vi "UART_U8Read_Timeout.vi"(8 "error in (no error)":errorcluster caption="错误输入（无错误）", 9 "断帧时间ms":u32=10, 10 "超时s":dbl=0.1, 11 "BASE_COM":refnum<visa-resource-name>="COM1") -> (0 "error out":errorcluster caption="错误输出", 1 "HasDat":bool, 2 "Strout":string, 3 "BASE_COM_OUT":refnum<visa-resource-name>)   [LabVIEW 2015, in "UARTCOM.lvlib"]
uses:
  UARTCOM.lvlib
panel:
  # ">=10ms"
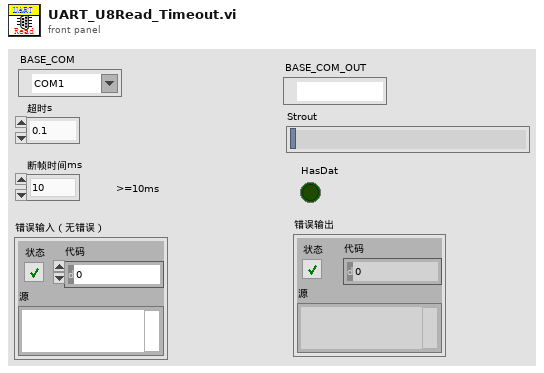
[diagram p1: front panel]
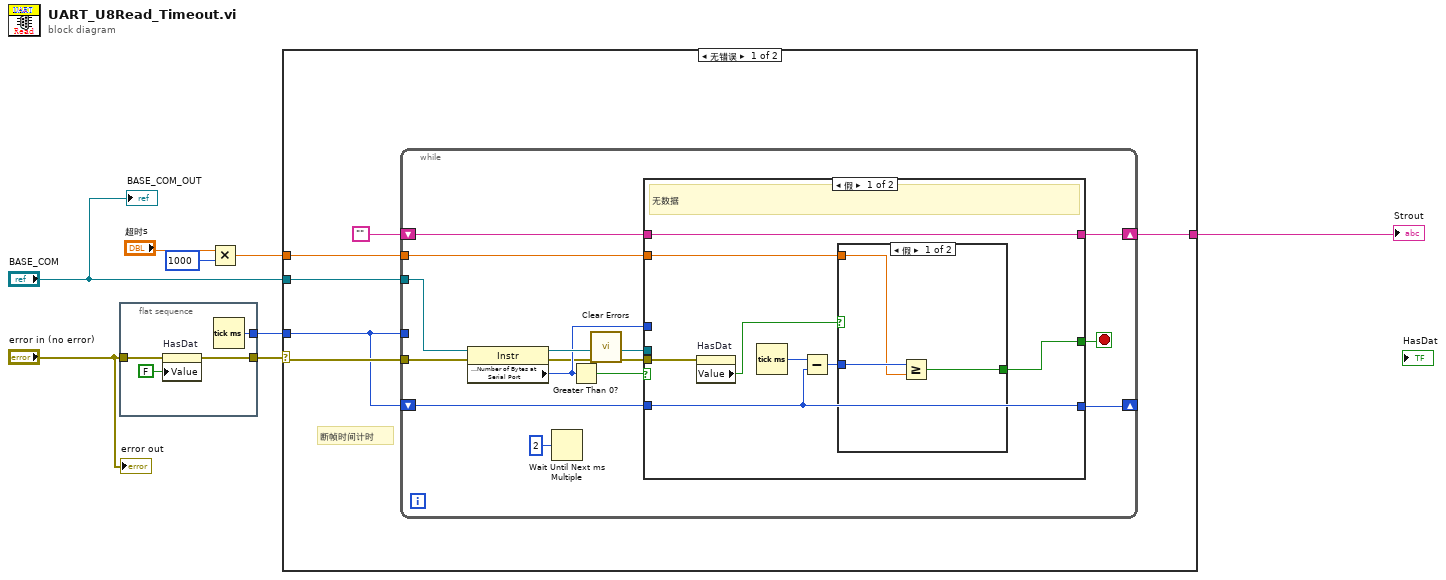
[diagram p0: block diagram]
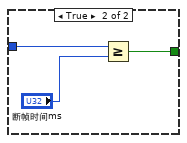
[diagram p2: hidden frame]
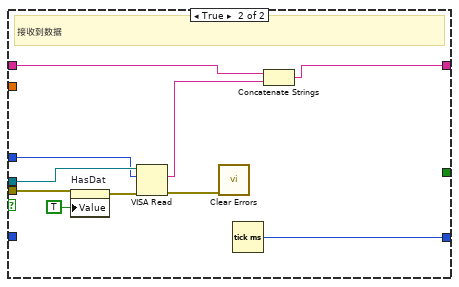
[diagram p3: hidden frame]
diagram:
  n1 = flat-sequence {
    tunnel: "error in (no error)" -> [w11]
    tunnel: [w10] -> w8
    tunnel: [w12] -> w7
    frame #0 {
      n2 = property on="HasDat" class="Bool (严格)"(error in=w11, "Value"=FALSE ("FirstIn")) -> (error out=w10:errorcluster)  [unwired: 1 in, 1 out]
      n3 = Tick Count (ms)() -> (millisecond timer value=w12:u32)
    }
  }
  n4 = Multiply(x="超时s", y=1000) -> (x*y=w4:dbl)
  n5 = case shown="无错误" w8 {
    selector: w8 -> [w17 _]
    tunnel: "BASE_COM" -> [w18 _]
    tunnel: w7 -> [w13 _]
    tunnel: w4 -> [w15 _]
    tunnel: [w14 _] -> w1
    frame No Error {
      # "断帧时间计时"
      n6 = while {
        tunnel: w18 -> [w32]
        tunnel: w17 -> [w31]
        tunnel: w13 -> [_]
        shift-right: [w24] -> w14
        shift-left: "" -> [w27]
        shift-right: [w28] -> _
        shift-left: w13 -> [w29]
        tunnel: w15 -> [w23]
        stop <- w22 stop-if-true
        n7 = property class="Instr"(reference=w32, error in=w31) -> (reference out=w26:refnum<visa-resource-name>, error out=w21:errorcluster, "Serial Settings:Number of Bytes at Serial Port"=w25:u32)
        n8 = Wait Until Next ms Multiple(millisecond multiple=u32 2 ("毫秒倍数")) -> ()  [unwired: 1 out]
        n9 = Greater Than 0?(x=w25) -> (x > 0?=w30:bool)
        n10 = call <vilib>:"Clear Errors.vi"("error in (no error)"=w21) -> ("error out"=w20:errorcluster)  [unwired: 5 in, 1 out]
        n11 = case shown="假" w30 {
          tunnel: w20 -> [w37 w56]
          tunnel: w29 -> [w39 _]
          tunnel: [w39 w54] -> w28
          tunnel: w27 -> [w38 w49]
          tunnel: w26 -> [_ w52]
          tunnel: w25 -> [_ w51]
          tunnel: [w38 w47] -> w24
          tunnel: w23 -> [w34 _]
          tunnel: [w33 _] -> w22
          frame False {
            # "无数据"
            n12 = property on="HasDat" class="Bool (严格)"(error in=w37) -> ("Value"=w36:bool)  [unwired: 1 in, 2 out]
            n13 = Tick Count (ms)() -> (millisecond timer value=w40:u32)
            n14 = Subtract(x=w40, y=w39) -> (x-y=w35:u32)
            n15 = case shown="假" w36 {
              tunnel: w35 -> [w43 w46]
              tunnel: w34 -> [w42 _]
              tunnel: [w41 w44] -> w33
              frame False {
                n16 = Greater Or Equal?(x=w43, y=w42) -> (x >= y?=w41:bool)
              }
              frame True {
                n17 = Greater Or Equal?(x=w46, y="断帧时间ms") -> (x >= y?=w44:bool)
              }
            }
          }
          frame True {
            # "接收到数据"
            n18 = property on="HasDat" class="Bool (严格)"(error in=w56, "Value"=TRUE ("FirstIn")) -> (error out=w53:errorcluster)  [unwired: 1 in, 1 out]
            n19 = VISA Read(VISA resource name=w52, byte count=w51, error in (no error)=w53) -> (read buffer=w48:string, error out=w50:errorcluster)  [unwired: 2 out]
            n20 = call <vilib>:"Clear Errors.vi"("error in (no error)"=w50) -> ()  [unwired: 5 in, 2 out]
            n21 = Tick Count (ms)() -> (millisecond timer value=w54:u32)
            n22 = Concatenate Strings(w49, w48) -> (w47:string)
          }
        }
      }
    }
    frame Error {
    }
  }
  "Strout" <- w1
  "error out" <- "error in (no error)"
  "BASE_COM_OUT" <- "BASE_COM"
